vi "HeadingCalc.vi"(10 "Target":dbl, 11 "Current":dbl) -> (3 "Dis&Dir":dbl)   [LabVIEW 2017]
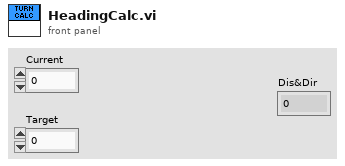
[diagram p1: front panel]
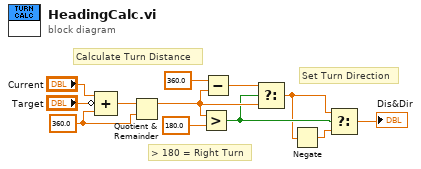
[diagram p0: block diagram]
diagram:
  w9 = 360.0 ("x")
  # "Set Turn Direction"
  # "> 180 = Right Turn"
  # "Calculate Turn Distance"
  n1 = Compound Arithmetic op=ADD("Current", invert "Target", w9) -> (w11:dbl)
  n2 = Quotient & Remainder(x=w11, y=w9) -> (x-y*floor(x/y)=w6:dbl)  [unwired: 1 out]
  n3 = Greater?(x=w6, y=180.0) -> (0:w4:bool)
  n4 = Subtract(x=360.0, y=w6) -> (x-y=w7:dbl)
  n5 = Select(t=w7, s=w4, f=w6) -> (s? t:f=w3:dbl)
  n6 = Negate(x=w3) -> (-x=w2:dbl)
  n7 = Select(t=w3, s=w4, f=w2) -> (s? t:f=→"Dis&Dir":dbl)
